vi "Evaluate Part 2.vi"() -> ()   [LabVIEW 2021]
uses:
  Proto/Module.lvclass
panel:
  out "delimited string":string
  out "Button presses":u64
  in  "Input":string
  # "2532512431 too high"
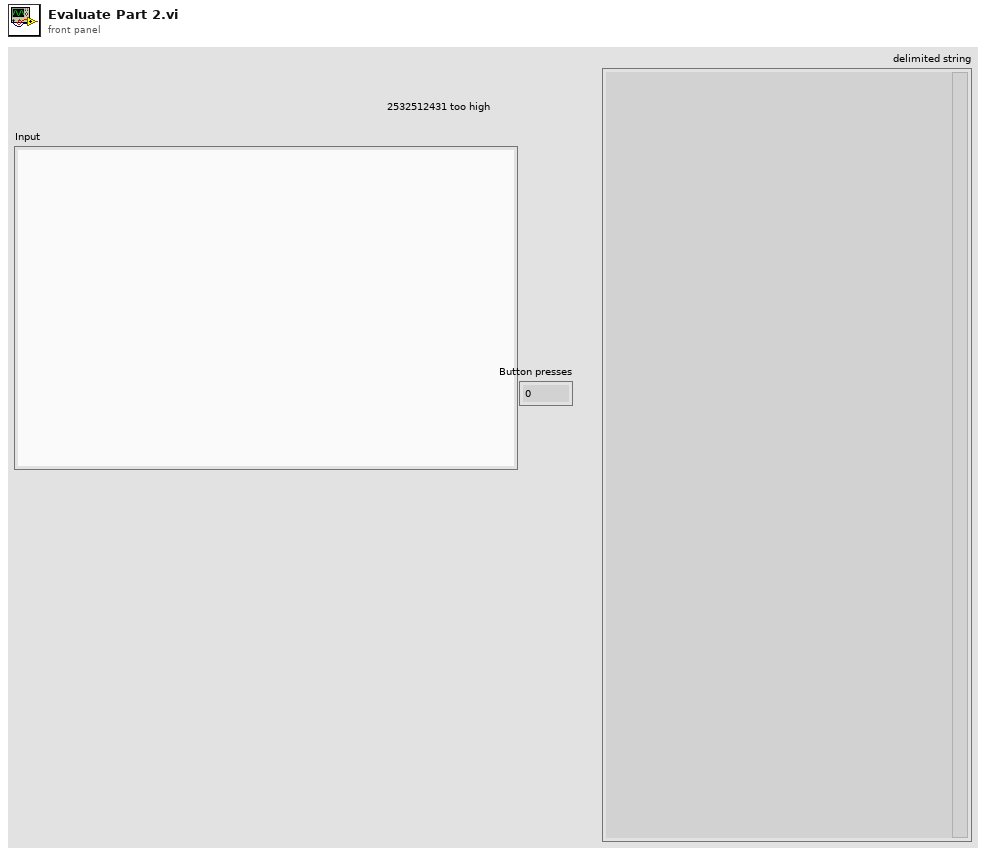
[diagram p1: front panel]
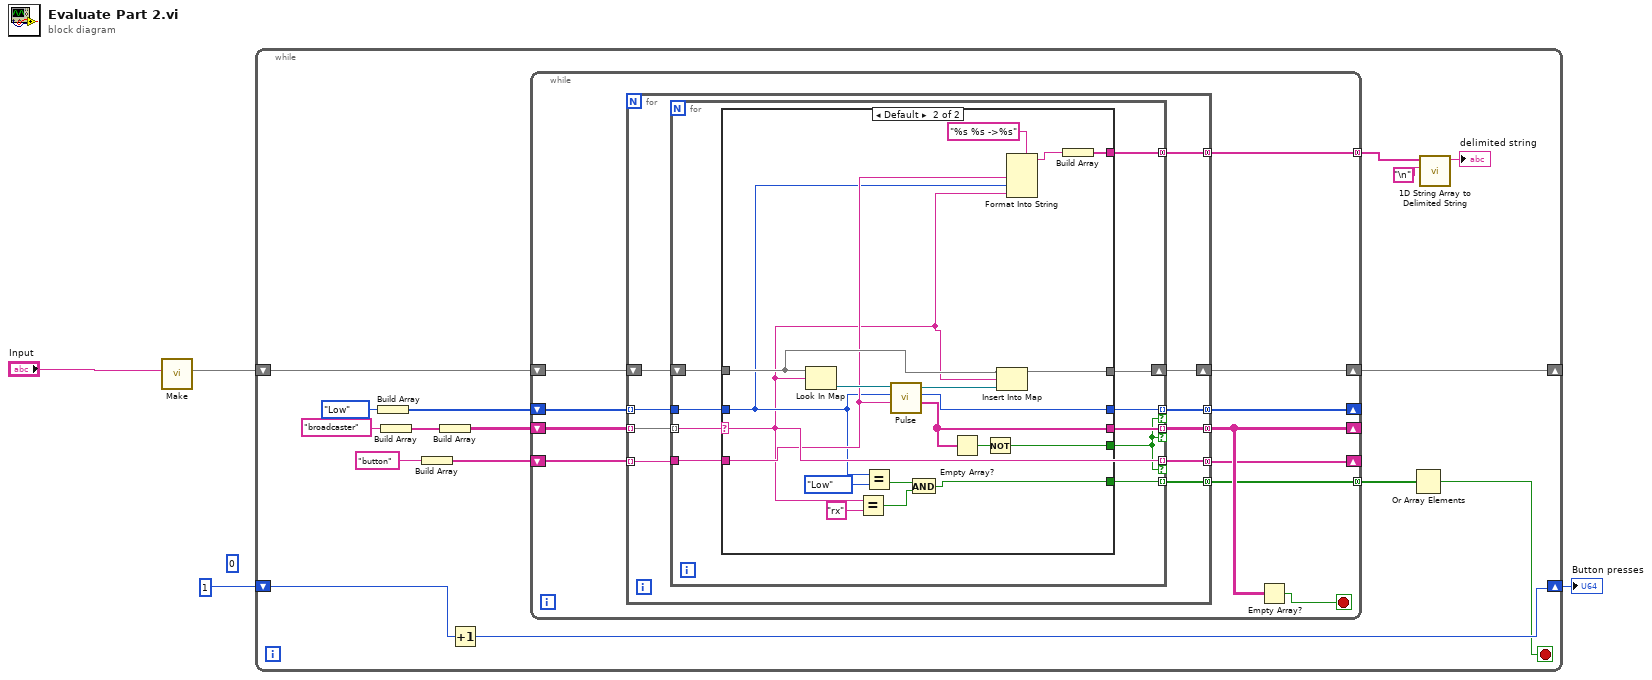
[diagram p0: block diagram]
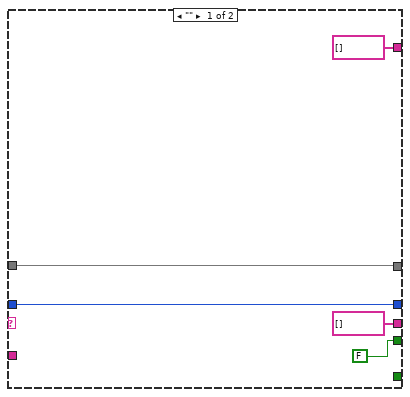
[diagram p2: hidden frame]
diagram:
  (unwired) u64 0
  n1 = call "Make.vi"("Input"="Input") -> ("map"=w4:map{string, refnum<class "Module.lvclass">})  [unwired: 8 in, 2 out]
  n2 = while {
    shift-right: [w12] -> _
    shift-left: w4 -> [w20]
    shift-right: [w9] -> w1
    shift-left: u64 1 -> [w10]
    stop <- w8 stop-if-true
    n3 = Build Array(enum16{"Low", "High"}."Low" ("Pulse In")) -> (w15:enum16{"Low", "High"}[])
    n4 = Build Array("broadcaster" ("key")) -> (w17:string[])
    n5 = Build Array("button" ("Sender")) -> (w14:string[])
    n6 = Build Array(w17) -> (w13:string[][])
    n7 = Increment(x=w10) -> (x+1=w9:u64)
    n8 = while {
      shift-right: [w26] -> _
      shift-left: w13 -> [w29]
      shift-right: [w27] -> _
      shift-left: w15 -> [w30]
      shift-right: [w25] -> _
      shift-left: w14 -> [w28]
      shift-right: [w24] -> w12
      shift-left: w20 -> [w31]
      tunnel: [w22] -> w11 mode=concatenating
      tunnel: [w21] -> w5 mode=concatenating
      stop <- w23 stop-if-true
      n9 = for {
        tunnel: w29 -> [w41] mode=indexing
        tunnel: w30 -> [w39] mode=indexing
        tunnel: [w38] -> w26 mode=concatenating
        tunnel: [w36] -> w27 mode=concatenating
        tunnel: w28 -> [w37] mode=indexing
        tunnel: [w35] -> w25 mode=concatenating
        shift-right: [w34] -> w24
        shift-left: w31 -> [w40]
        tunnel: [w33] -> w22 mode=concatenating
        tunnel: [w32] -> w21 mode=concatenating
        n10 = for {
          tunnel: w41 -> [w46] mode=indexing
          tunnel: [w45] -> w38 mode=indexing if=w44
          tunnel: w37 -> [w49]
          tunnel: [w46] -> w35 mode=indexing if=w44
          shift-right: [w47] -> w34
          shift-left: w40 -> [w48]
          tunnel: w39 -> [w50]
          tunnel: [w51] -> w36 mode=indexing if=w44
          tunnel: [w43] -> w33 mode=indexing
          tunnel: [w42] -> w32 mode=concatenating
          n11 = case shown="Default" w46 {
            selector: w46 -> [_ w58]
            tunnel: [w55 w74] -> w51
            tunnel: w50 -> [w55 w59]
            tunnel: w49 -> [_ w60]
            tunnel: w48 -> [w56 w73]
            tunnel: [w56 w72] -> w47
            tunnel: [string[] [] ("Receivers") w70] -> w45
            tunnel: [FALSE w68] -> w44
            tunnel: [_ w63] -> w43
            tunnel: [string[] [] w57] -> w42
            frame "" {
            }
            frame Default {
              n12 = Look In Map(map=w73, key=w58) -> (value=w75:refnum<class "Module.lvclass">)  [unwired: 1 in, 1 out]
              n13 = Equal?(x=w58, y="rx") -> (x = y?=w64:bool)
              n14 = Equal?(x=w59, y=enum16{"Low", "High"}."Low") -> (x = y?=w65:bool)
              n15 = call-dynamic "Pulse.vi"("Sender"=w60, "Pulse In"=w59, "Module In"=w75) -> ("Receivers"=w70:string[], "Pulse Out"=w74:enum16{"Low", "High"}, "Module Out"=w71:refnum<class "Module.lvclass">)  [unwired: 5 in, 1 out]
              n16 = And(x=w65, y=w64) -> (x .and. y?=w63:bool)
              n17 = Empty Array?(array=w70) -> (empty?=w69:bool)
              n18 = Not(x=w69) -> (.not. x?=w68:bool)
              n19 = Insert Into Map(map in=w73, key=w58, value=w71) -> (map out=w72:map{string, refnum<class "Module.lvclass">})  [unwired: 2 out]
              n20 = Format Into String(format string="%s %s ->%s", w60, w59, w58) -> (resulting string=w62:string)  [unwired: 2 in, 1 out]
              n21 = Build Array(w62) -> (w57:string[])
            }
          }
        }
      }
      n22 = Empty Array?(array=w26) -> (empty?=w23:bool)
    }
    n23 = Or Array Elements(Boolean array=w11) -> (logical OR=w8:bool)
    n24 = call <vilib>:"1D String Array to Delimited String.vi"("delimiter"="\n", "string array"=w5) -> ("delimited string"=→"delimited string":string)  [unwired: 9 in]
  }
  "Button presses" <- w1
